vi "Assign07_MECE301_Simulator.vi"() -> (3 "Color":T1(ring))   [LabVIEW 2013]
doc: "This VI simulates an acquisition by randomly providing one of six colors of m&m's: red, blue, green, yellow, brown, or orange. The acquisition rate is simulated at 50 msec for each measurement cycle.\n\nJohn D. Wellin\nSenior Lecturer\nDept. of Mechanical Engineering\nJames E. Gleason Bldg. 09-2014\n76 Lomb Memorial Drive\nRochester, NY 14623\nOffice: 585-475-5223\nFax: 585-475-7710\nE-mail: jdweme@rit.edu"
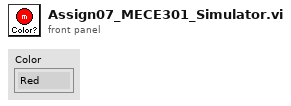
[diagram p1: front panel]
types:
  T1 = enum16{"Red", "Blue", "Green", "Yellow", "Brown", "Orange"}
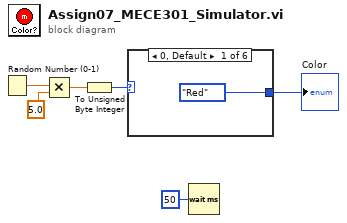
[diagram p0: block diagram]
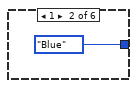
[diagram p2: hidden frame]
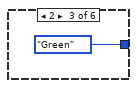
[diagram p3: hidden frame]
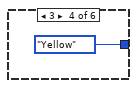
[diagram p4: hidden frame]
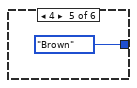
[diagram p5: hidden frame]
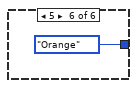
[diagram p6: hidden frame]
diagram:
  n1 = Random Number (0-1)() -> (number: 0 to 1=w6:dbl)
  n2 = Multiply(x=w6, y=5.0) -> (x*y=w4:dbl)
  n3 = To Unsigned Byte Integer(number=w4) -> (unsigned 8bit integer=w2:u8)
  n4 = case shown="0, Default" w2 {
    tunnel: [T1."Red" T1."Blue" T1."Green" T1."Yellow" T1."Brown" T1."Orange"] -> w1
    frame 0, Default {
    }
    frame 1 {
    }
    frame 2 {
    }
    frame 3 {
    }
    frame 4 {
    }
    frame 5 {
    }
  }
  "Color" <- w1
  n5 = Wait (ms)(milliseconds to wait=u32 50) -> ()  [unwired: 1 out]
